vi "Open.vi"(8 "error in (no error)":errorcluster, 11 "Device":refnum<class "Device.lvclass">) -> (0 "error out":errorcluster, 3 "RTL-SDR out":refnum<class "Session.lvclass">)   [LabVIEW 2020, in "RTL-SDR.lvlib" / "Session.lvclass"]
uses:
  Session.lvclass
  Device/Device.lvclass
  Session.lvclass/Session.ctl
  lib/librtlsdr.dll
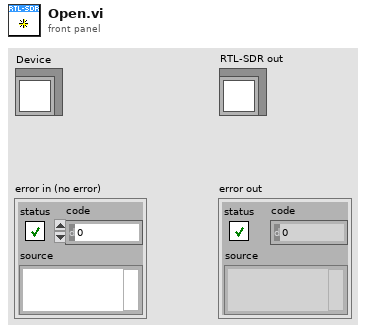
[diagram p1: front panel]
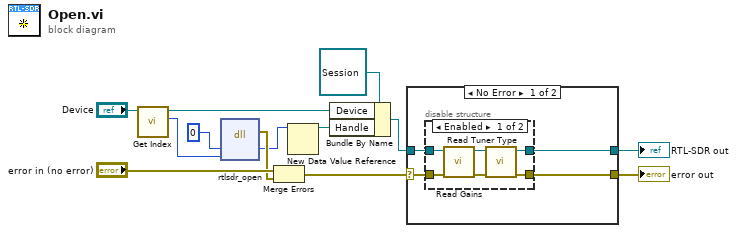
[diagram p0: block diagram]
diagram:
  n1 = call "Get Index.vi"("Device in"="Device") -> ("Index"=w9:u32, "Device out"=w10:refnum<class "Device.lvclass">)  [unwired: 8 in, 1 out]
  n2 = dll-call lib="C:/dev/IlluminatedG/lv-rtl-sdr/lib/librtlsdr.dll" fn="rtlsdr_open"("dev"=u64 0, "index"=w9) -> (error out=w7:errorcluster, "dev"=w2:u64)  [unwired: 5 in, 1 out]
  n3 = Merge Errors("error in (no error)", w7) -> (w6:errorcluster)
  n4 = New Data Value Reference(data value=w2) -> (data value reference=w1:refnum<data-value>)  [unwired: 1 in, 1 out]
  n5 = Bundle By Name(cluster=refnum<class "Session.lvclass"> refnum ("RTL-SDR in"), "Device"=w10, "Handle"=w1) -> (w5:refnum<class "Session.lvclass">)
  n6 = case shown="No Error" w6 {
    selector: w6 -> [w17 w26]
    tunnel: w5 -> [w16 w27]
    tunnel: [w15 w26] -> w4
    tunnel: [w14 w27] -> w3
    frame No Error {
      n7 = disable-structure shown="Enabled" {
        disable-tunnel: w17 -> [w23 w25]
        disable-tunnel: w16 -> [w22 w24]
        disable-tunnel: [w19 w25] -> w15
        disable-tunnel: [w18 w24] -> w14
        frame Enabled {
          n8 = call "Read Gains.vi"("error in (no error)"=w23, "RTL-SDR in"=w22) -> ("error out"=w20:errorcluster, "RTL-SDR out"=w21:refnum<class "Session.lvclass">)  [unwired: 8 in]
          n9 = call "Read Tuner Type.vi"("error in (no error)"=w20, "RTL-SDR in"=w21) -> ("error out"=w19:errorcluster, "RTL-SDR out"=w18:refnum<class "Session.lvclass">)  [unwired: 8 in]
        }
        frame Disabled {
        }
      }
    }
    frame Error {
    }
  }
  "error out" <- w4
  "RTL-SDR out" <- w3
